vi "Write Golf Club.vi"(8 "error in (no error)":errorcluster, 10 "Golf Club.lvclass":refnum<class "Golf Club.lvclass">, 11 "Bill Murray in":refnum<class "Bill Murray.lvclass">) -> (0 "error out":errorcluster, 3 "Bill Murray out":refnum<class "Bill Murray.lvclass">)   [LabVIEW 2019, in "Bill Murray.lvclass"]
uses:
  Bill Murray.lvclass
  Golf Club.lvclass
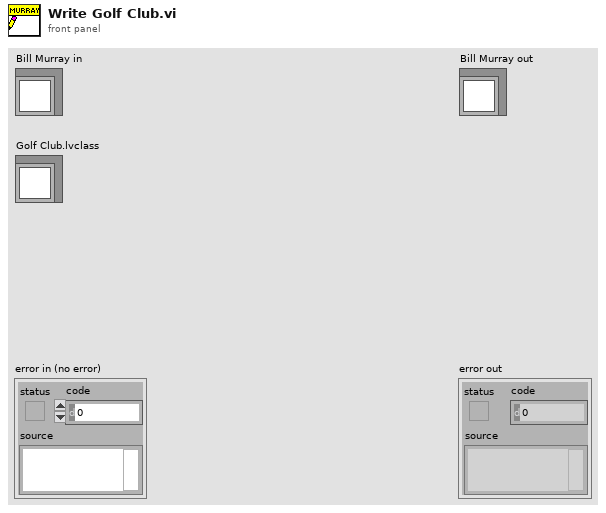
[diagram p1: front panel]
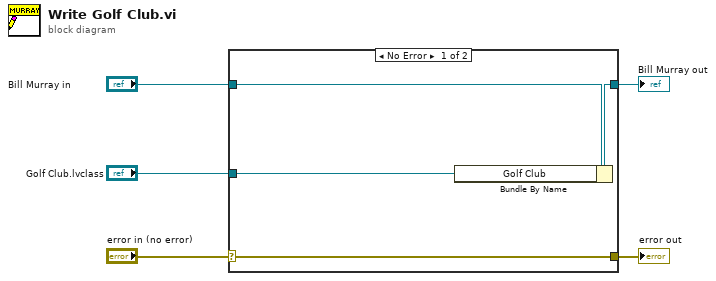
[diagram p0: block diagram]
diagram:
  n1 = case shown="No Error" "error in (no error)" {
    selector: "error in (no error)" -> [w9 w10]
    tunnel: [w9 w10] -> w4
    tunnel: [w7 w11] -> w2
    tunnel: "Bill Murray in" -> [w8 w11]
    tunnel: "Golf Club.lvclass" -> [w6 _]
    frame No Error {
      n2 = Bundle By Name(cluster=w8, "Golf Club"=w6) -> (w7:refnum<class "Bill Murray.lvclass">)
    }
    frame Error {
    }
  }
  "error out" <- w4
  "Bill Murray out" <- w2
